vi "delRepArgVar.vi"(11 "sec+*var":string[](array[string])) -> (1 "sec":string, 2 "*varNoRepeatArr":string[](array[string]), 3 "sec+*varNoRepeatArr":string[](array[string]))   [LabVIEW 2010]
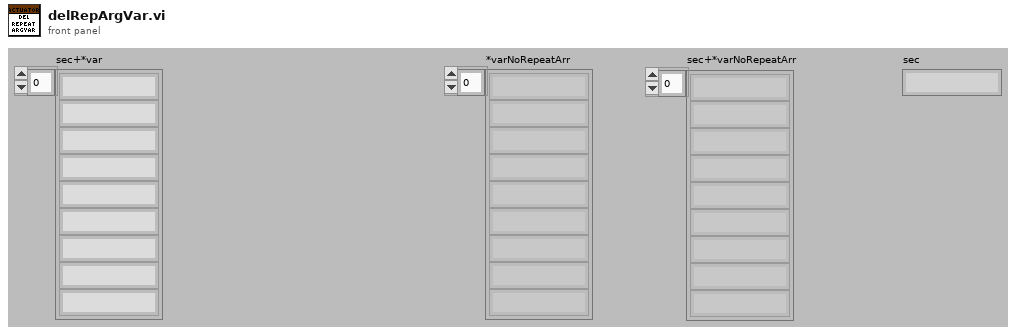
[diagram p1: front panel]
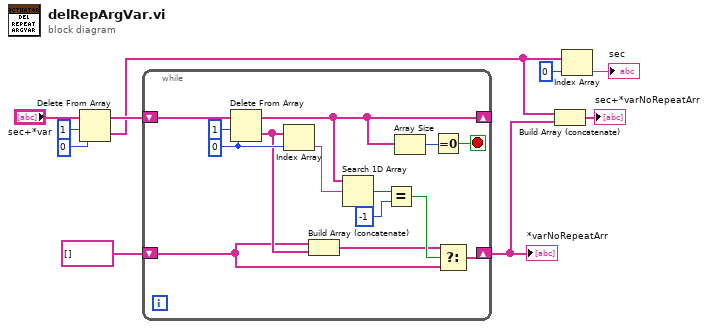
[diagram p0: block diagram]
diagram:
  n1 = Delete From Array(array="sec+*var", length=1 ("index"), index=0) -> (deleted portion=w3:string[], array with subset deleted=w7:string[])
  n2 = while {
    shift-right: [w13] -> _
    shift-left: w7 -> [w23]
    shift-right: [w14] -> w6
    shift-left: string[] [] -> [w15]
    stop <- w11 stop-if-true
    w22 = 0 ("index")
    n3 = Delete From Array(array=w23, length=1, index=w22) -> (deleted portion=w17:string[], array with subset deleted=w13:string[])
    n4 = Index Array(array=w17, index=w22) -> (element=w21:string)
    n5 = Build Array (concatenate)(w15, w17) -> (w16:string[])
    n6 = Search 1D Array(1D array=w13, element=w21) -> (index of element=w20:i32)  [unwired: 1 in]
    n7 = Equal?(x=w20, y=-1) -> (x = y?=w18:bool)
    n8 = Array Size(array=w13) -> (size(s)=w12:i32)
    n9 = Equal To 0?(x=w12) -> (x = 0?=w11:bool)
    n10 = Select(t=w16, s=w18, f=w15) -> (s? t:f=w14:string[])
  }
  "*varNoRepeatArr" <- w6
  n11 = Build Array (concatenate)(w3, w6) -> (→"sec+*varNoRepeatArr":string[])
  n12 = Index Array(array=w3, index=0) -> (element=→"sec":string)
